vi "NewtonSolverForSquareFunctions.vi"(0 "a":dbl, 1 "x lower bound":dbl, 5 "b":dbl, 7 "c":dbl, 9 "d":dbl, 11 "x_0":dbl, 12 "x upper bound":dbl) -> (15 "x_n":dbl)   [LabVIEW 2021]
panel:
  # "f''(x)+"
  # "f'(x)+"
  # "f(x)+"
  # "= 0"
  # "<x<"
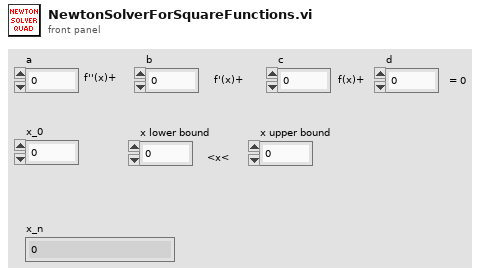
[diagram p1: front panel]
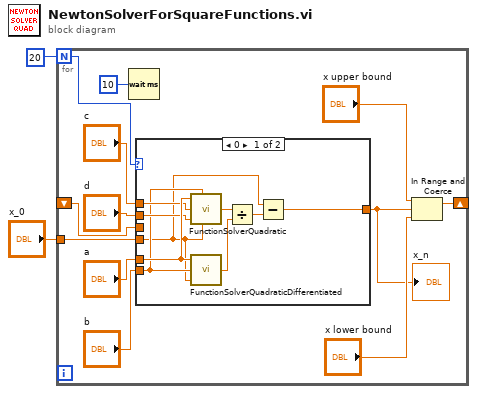
[diagram p0: block diagram]
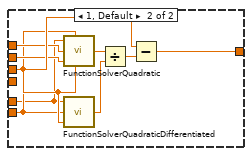
[diagram p2: hidden frame]
diagram:
  n1 = for {
    N: 20 -> [w3]
    shift-right: [w5] -> _
    shift-left: _ -> [w14]
    tunnel: "x_0" -> [w8]
    n2 = Wait (ms)(milliseconds to wait=u32 10) -> ()  [unwired: 1 out]
    n3 = case shown="0" w3 {
      tunnel: [w15 w32] -> w4
      tunnel: w14 -> [_ w28]
      tunnel: "d" -> [w18 w27]
      tunnel: "c" -> [w19 w26]
      tunnel: "b" -> [w17 w25]
      tunnel: "a" -> [w20 w24]
      tunnel: w8 -> [w16 _]
      frame 0 {
        n4 = call "FunctionSolverQuadratic.vi"("a"=w20, "b"=w17, "c"=w19, "d"=w18, "x"=w16) -> ("f(x)"=w23:dbl)
        n5 = call "FunctionSolverQuadraticDifferentiated.vi"("x"=w16, "b"=w17, "a"=w20) -> ("f'(x)"=w22:dbl)
        n6 = Divide(x=w23, y=w22) -> (x/y=w21:dbl)
        n7 = Subtract(x=w16, y=w21) -> (x-y=w15:dbl)
      }
      frame 1, Default {
        n8 = call "FunctionSolverQuadratic.vi"("a"=w24, "b"=w25, "c"=w26, "d"=w27, "x"=w28) -> ("f(x)"=w31:dbl)
        n9 = call "FunctionSolverQuadraticDifferentiated.vi"("x"=w28, "b"=w25, "a"=w24) -> ("f'(x)"=w30:dbl)
        n10 = Divide(x=w31, y=w30) -> (x/y=w29:dbl)
        n11 = Subtract(x=w28, y=w29) -> (x-y=w32:dbl)
      }
    }
    "x_n" <- w4
    n12 = In Range and Coerce(upper limit="x upper bound", x=w4, lower limit="x lower bound") -> (coerced(x)=w5:dbl)  [unwired: 1 out]
  }
